vi "Do.vi"(8 "error in (no error)":errorcluster, 10 "Actor in":refnum<class "Actor.lvclass">, 11 "Endpoint Connected Msg":refnum<class "Endpoint Connected Msg.lvclass">) -> (0 "error out":errorcluster, 2 "Actor out":refnum<class "Actor.lvclass">)   [LabVIEW 2019, in "Cobra RT.lvlib" / "Endpoint Connected Msg.lvclass"]
doc: "This VI delivers the message to the actor by calling the appropriate method(s) on the actor."
uses:
  Endpoint Connected Msg.lvclass
  C:/Program Files (x86)/National Instruments/LabVIEW 2019/vi.lib/ni/Actors/Network Endpoint Actors/Nested Endpoint/Nested Endpoint Messages/Connected Msg/Connected Msg.lvclass
  <vilib>/ActorFramework/Actor/Actor.lvclass
  Cobra RT/Cobra RT.lvclass
  C:/Program Files (x86)/National Instruments/LabVIEW 2019/vi.lib/ActorFramework/Actor/Actor.lvclass
  <vilib>/ni/Actors/Network Endpoint Actors/Nested Endpoint/Nested Endpoint Messages/Connected Msg/Connected Msg.lvclass/Connected Msg.ctl
  <vilib>/ni/Actors/Network Endpoint Actors/Nested Endpoint/Nested Endpoint Messages/Connected Msg/Connected Msg.lvclass
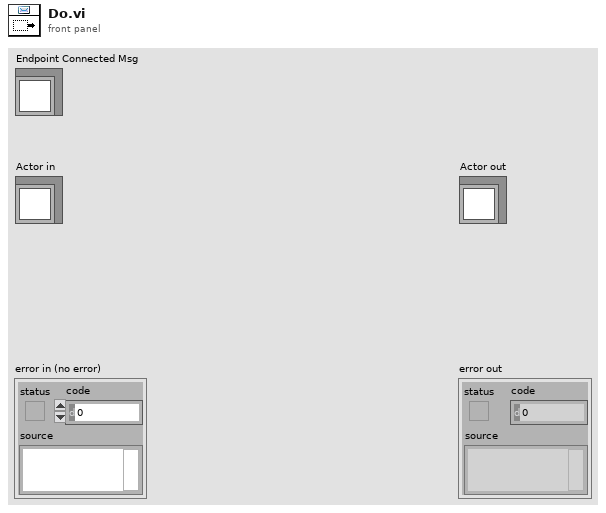
[diagram p1: front panel]
types:
  T1 = cluster{"Endpoint Enqueuer":refnum<class "Message Enqueuer.lvclass">}
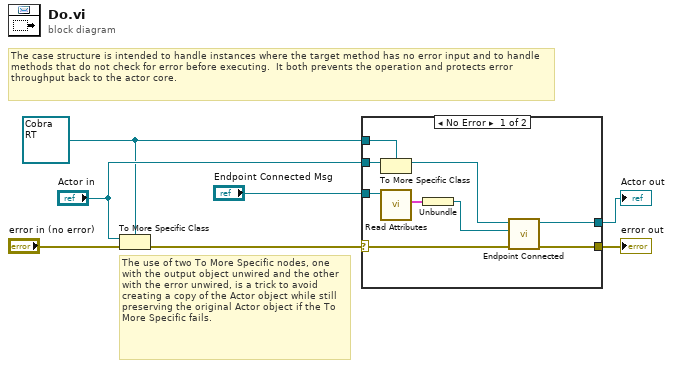
[diagram p0: block diagram]
diagram:
  w1 = refnum<class "Cobra RT.lvclass"> refnum ("Cobra RT.lvlib:Cobra RT.lvclass")
  # "The use of two To More Specific nodes, one with the output object unwired and the other with the error unwired, is a trick to avoid creating a copy of the Actor object while still preserving the original Actor object if the To More Specific fails."
  # "The case structure is intended to handle instances where the target method has no error input and to handle methods that do not check for error before executing.  It both prevents the operation and protects error throughput back to the actor core."
  n1 = To More Specific Class(target class=w1, reference="Actor in", error in="error in (no error)") -> (error out=w6:errorcluster)  [unwired: 1 out]
  n2 = case shown="No Error" w6 {
    selector: w6 -> [w12 w18]
    tunnel: [w11 w18] -> w5
    tunnel: [w10 w17] -> w4
    tunnel: "Actor in" -> [w16 w17]
    tunnel: w1 -> [w15 _]
    tunnel: "Endpoint Connected Msg" -> [w13 _]
    frame No Error {
      n3 = To More Specific Class(target class=w15, reference=w16) -> (specific class reference=w8:refnum<class "Cobra RT.lvclass">)  [unwired: 1 in, 1 out]
      n4 = call <vilib>:"Read Attributes.vi"("Connected Msg"=w13) -> ("Payload"=w14:T1)  [unwired: 10 in]
      n5 = Unbundle(w14) -> ("Endpoint Enqueuer"=w9:refnum<class "Message Enqueuer.lvclass">)
      n6 = call "Endpoint Connected.vi"("error in (no error)"=w12, "Endpoint Enqueuer"=w9, "Cobra RT in"=w8) -> ("error out"=w11:errorcluster, "Cobra RT out"=w10:refnum<class "Cobra RT.lvclass">)  [unwired: 7 in]
    }
    frame Error {
      # "If type check fails, pass the original object out again."
    }
  }
  "error out" <- w5
  "Actor out" <- w4
